vi "Read Actor Ref.vi"(11 "Setup in":refnum<class "Setup.lvclass">) -> (2 "Actor Ref":refnum<vi>)   [LabVIEW 2025, in "jettl.lvlib" / "Setup.lvlib" / "Setup.lvclass"]
uses:
  Setup.lvclass
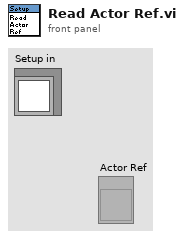
[diagram p1: front panel]
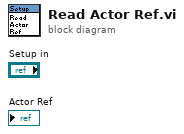
[diagram p0: block diagram]
diagram:
